vi "Intensity Chart dy.vi"(8 "Error In":errorcluster, 9 "Acqusition Result":T1={"Traces"=[], "Relative t0 [s]"=1000.0, "Sample Rate [1/s]"=1000.0, "No. of points"=0, "Absolute t0 [s]"=1000.0, "dT [s]"=1000.0, "Update rate [1/s]"=0.0, "Auto Triggered"=FALSE} {"Update rate [1/s]" format="%_3p"}, 11 "Intensity charts":refnum<vi>[](array[refnum])) -> (0 "Error Out":errorcluster, 3 "Intensity charts":refnum<vi>[](array[refnum]))   [LabVIEW 2017]
uses:
  Controls/Acquisition Result.ctl
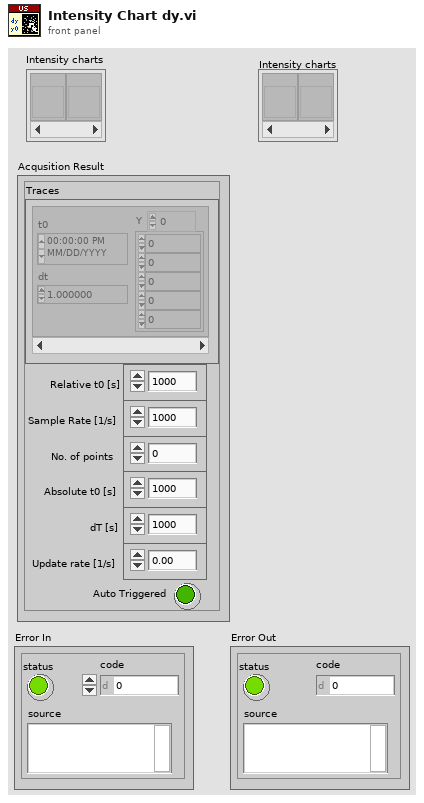
[diagram p1: front panel]
types:
  T1 = typedef "Acquisition Result.ctl" = cluster{"Traces":waveform(dbl)[], "Relative t0 [s]":dbl, "Sample Rate [1/s]":dbl, "No. of points":i32, "Absolute t0 [s]":dbl, "dT [s]":dbl, "Update rate [1/s]":dbl, "Auto Triggered":bool}
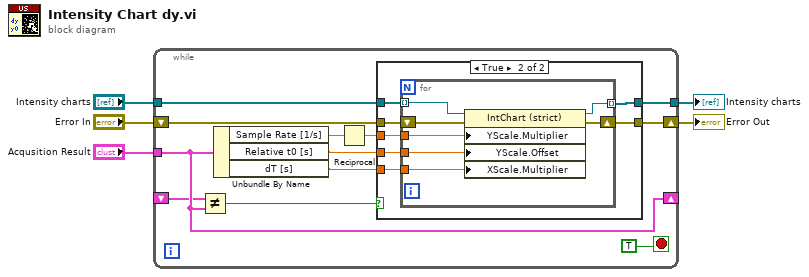
[diagram p0: block diagram]
diagram:
  n1 = while {
    tunnel: "Intensity charts" -> [w17]
    shift-right: [w16] -> w4
    shift-left: "Error In" -> [w15]
    shift-right: [w7] -> _
    shift-left: _ -> [w6]
    tunnel: [w13] -> w2
    tunnel: "Acqusition Result" -> [w7]
    stop <- TRUE stop-if-true
    n2 = Not Equal?(x=w6, y=w7) -> (x != y?=w12:bool)
    n3 = Unbundle By Name(w7) -> ("Sample Rate [1/s]"=w11:dbl, "Relative t0 [s]"=w9:dbl, "dT [s]"=w8:dbl)
    n4 = Reciprocal(x=w11) -> (1/x=w10:dbl)
    n5 = case shown="True" w12 {
      tunnel: w17 -> [w18 w26]
      tunnel: [w19 w25] -> w16
      tunnel: w15 -> [w19 w24]
      tunnel: w10 -> [_ w23]
      tunnel: w9 -> [_ w22]
      tunnel: [w18 w21] -> w13
      tunnel: w8 -> [_ w20]
      frame False {
      }
      frame True {
        n6 = for {
          tunnel: w26 -> [w33] mode=indexing
          tunnel: w23 -> [w31]
          shift-right: [w32] -> w25
          shift-left: w24 -> [w30]
          tunnel: w22 -> [w29]
          tunnel: [w28] -> w21 mode=indexing
          tunnel: w20 -> [w27]
          n7 = property class="IntChart (strict)"(reference=w33, error in=w30, "YScale.Multiplier"=w31, "YScale.Offset"=w29, "XScale.Multiplier"=w27) -> (reference out=w28:refnum<vi>, error out=w32:errorcluster)
        }
      }
    }
  }
  "Error Out" <- w4
  "Intensity charts" <- w2
